vi "swerve_periodic.vi"(8 "Field Oriented?":bool, 9 "Rotate":dbl(slide) scale=-1.0..1.0, 10 "Forwards":dbl(slide) scale=-1.0..1.0, 11 "Strafe":dbl(slide) scale=-1.0..1.0) -> ()   [LabVIEW 2020]
uses:
  <vilib>/Rock Robotics/WPI/ThirdParty/Phoenix-LabVIEW/Motor Controller/Controls/CTRE_Phoenix_MotorControl_ControlMode.ctl
  swerve_globals.vi
  <vilib>/Rock Robotics/WPI/ThirdParty/Phoenix-LabVIEW/Motor Controller/Get/CTRE_Phoenix_MotorController_GetSelectedSensorData.vi
  TitanLib/Lib/TitanLib.lvlib
panel:
  in  "Set Constants":bool
  in  "Constants":T1
  out "Pose Estimation (in)":cluster{"Pose[0]":dbl, "Pose[1]":dbl}[](graph)
  in  "wheel offset (in)":dbl format="%_6g"
  in  "Reset Odometry?":bool
  in  "Drive Speed Multiplier":dbl=1.0
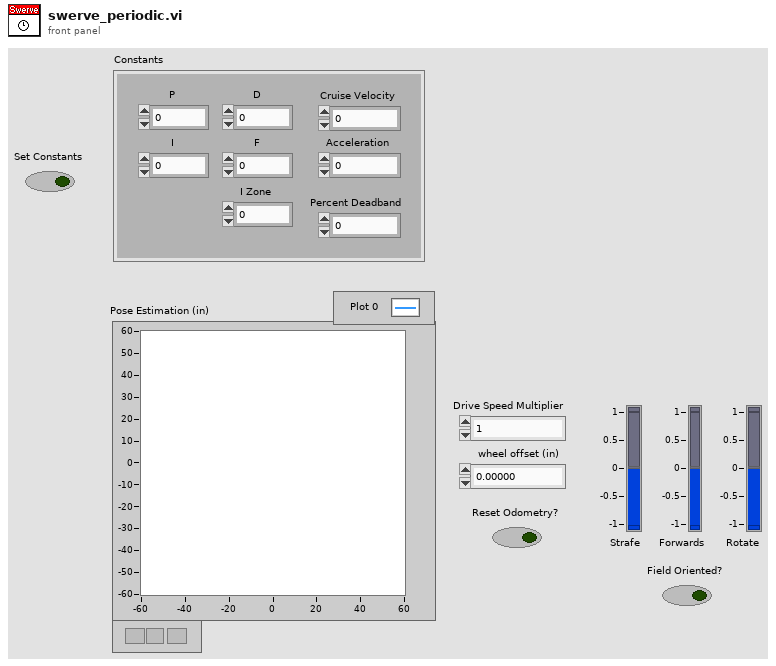
[diagram p1: front panel]
types:
  T1 = cluster{"P":dbl, "I":dbl, "D":dbl, "F":dbl, "I Zone":dbl, "Cruise Velocity":i32, "Acceleration":i32, "Percent Deadband":dbl}
  T2 = typedef "CTRE_Phoenix_MotorControl_ControlMode.ctl" = u16
  T3 = typedef "WPI_MotorControlDeviceRef.ctl" = cluster{"DeviceStatus":errorcluster, "Type":T4, "PWM":cluster{"PWM Channel":T5, "DeadBand":T6}, "CAN":cluster{"Device Number":u8, "SetOutput VI Ref":variant, "GetOutput VI Ref":variant, "Enable VI Ref":variant, "Disable VI Ref":variant, "Data":variant}, "Invert":bool, "DIO PWM":cluster{"PWM \"Enable\" Channel":T5, "DIOChannel":T7, "PWM Rate":dbl}}
  T4 = typedef "WPI_MotorControlType.ctl" = enum16{"PWM", "CAN", "DIO PWM"}
  T5 = typedef "FPGA_DIOPWMChannel.ctl" = enum8{"PWM 0", "PWM 1", "PWM 2", "PWM 3", "PWM 4", "PWM 5", "PWM 6", "PWM 7", "PWM 8", "PWM 9", "PWM MXP 0", "PWM MXP 1", "PWM MXP 2", "PWM MXP 3", "PWM MXP 4", "PWM MXP 5", "PWM MXP 6", "PWM MXP 7", "PWM MXP 8", "PWM MXP 9", "Invalid"}
  T6 = typedef "WPI_PWMDeadband.ctl" = cluster{"Name":string, "maxPositivePwm":i32, "minPositivePwm":i32, "centerPwm":i32, "maxNegativePwm":i32, "minNegativePwm":i32, "angularRange":u16}
  T7 = typedef "FPGA_DIOChannel.ctl" = enum8{"DIO 0", "DIO 1", "DIO 2", "DIO 3", "DIO 4", "DIO 5", "DIO 6", "DIO 7", "DIO 8", "DIO 9", "DIO MXP 0", "DIO MXP 1", "DIO MXP 2", "DIO MXP 3", "DIO MXP 4", "DIO MXP 5", "DIO MXP 6", "DIO MXP 7", "DIO MXP 8", "DIO MXP 9", "DIO MXP 10", "DIO MXP 11", "DIO MXP 12", "DIO MXP 13", "DIO MXP 14", "DIO MXP 15", "SPI Port CS1", "SPI Port CS2", "SPI Port CS3", "SPI Port MISO", "SPI Port MOSI", "Invalid"}
  T8 = typedef "NI_Matrix.lvlib/RealMatrix.ctl" = dbl[][]
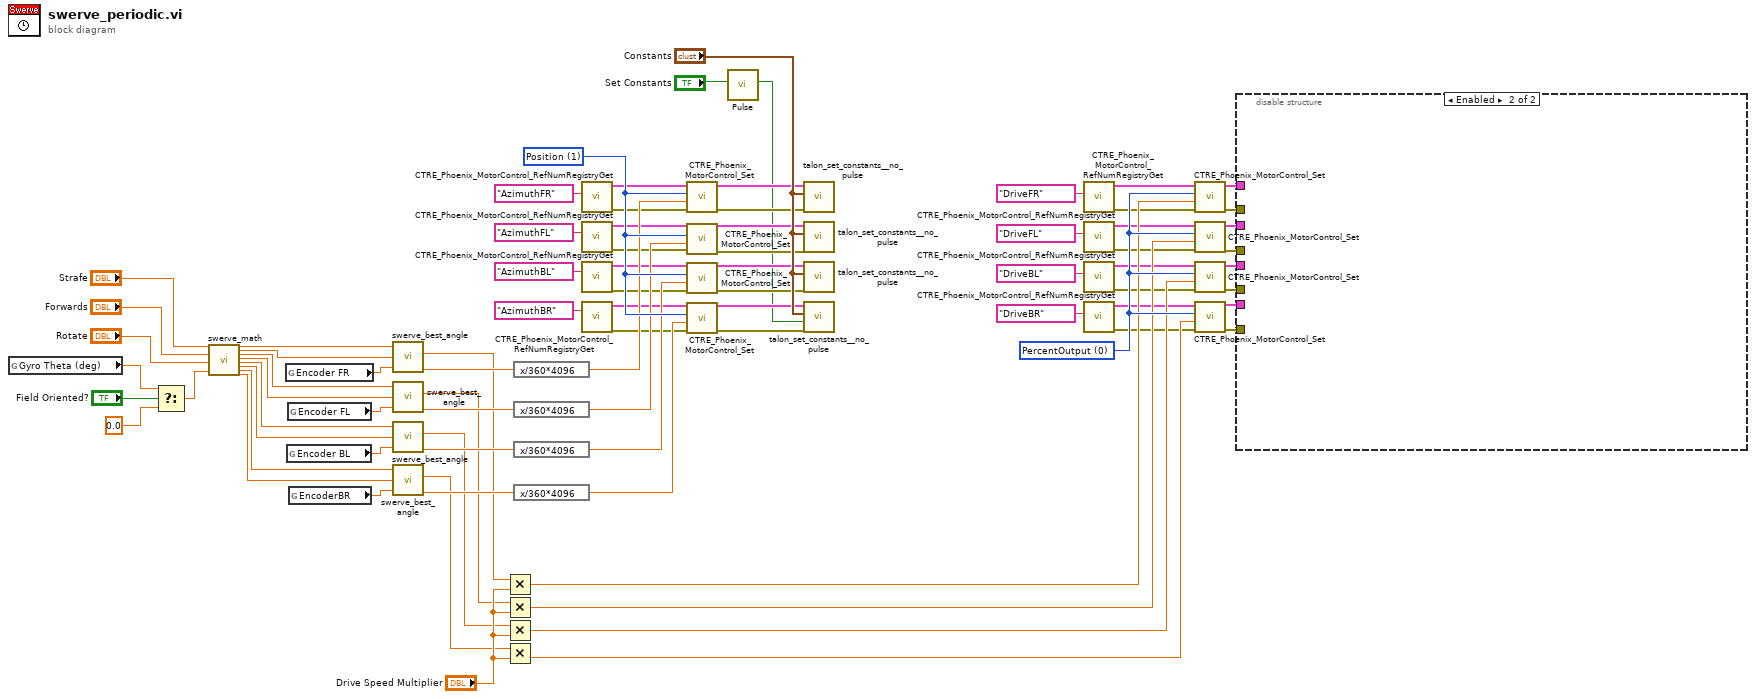
[diagram p0: block diagram]
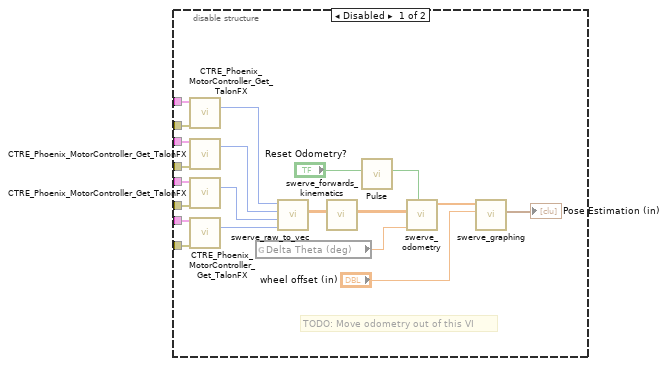
[diagram p2: hidden frame]
diagram:
  w67 = T2 0 items=["PercentOutput"=0, "Position"=1, "Velocity"=2, "Current"=3, "Follower"=5, "MotionProfile"=6, "MotionMagic"=7, "MotionProfileArc"=10, "Disabled"=15] ("Control Mode")
  w81 = T2 1 items=["PercentOutput"=0, "Position"=1, "Velocity"=2, "Current"=3, "Follower"=5, "MotionProfile"=6, "MotionMagic"=7, "MotionProfileArc"=10, "Disabled"=15] ("Control Mode")
  n1 = global read "swerve_globals.vi" "Gyro Theta (deg)"() -> (w18:dbl)
  n2 = Select(t=w18, s="Field Oriented?", f=0.0) -> (s? t:f=w16:dbl)
  n3 = call "swerve_math.vi"("Strafe"="Strafe", "Forwards"="Forwards", "Rotate"="Rotate", "Gyro"=w16) -> ("Drive FR"=w30:dbl, "Azimuth FR"=w25:dbl, "Drive FL"=w24:dbl, "Azimuth FL"=w23:dbl, "Drive BL"=w22:dbl, "Azimuth BL"=w21:dbl, "Drive BR"=w20:dbl, "Azimuth BR"=w19:dbl)  [unwired: 16 in]
  n4 = global read "swerve_globals.vi" "Encoder FR"() -> (w29:dbl)
  n5 = global read "swerve_globals.vi" "Encoder BL"() -> (w27:dbl)
  n6 = global read "swerve_globals.vi" "Encoder FL"() -> (w28:dbl)
  n7 = global read "swerve_globals.vi" "EncoderBR"() -> (w26:dbl)
  n8 = call "swerve_best_angle.vi"("Current Angle"=w29, "Target Angle"=w25, "Power In"=w30) -> ("Setpoint Angle"=w80:dbl, "Power Out"=w71:dbl)  [unwired: 4 in]
  n9 = call "swerve_best_angle.vi"("Current Angle"=w28, "Target Angle"=w23, "Power In"=w24) -> ("Setpoint Angle"=w79:dbl, "Power Out"=w70:dbl)  [unwired: 4 in]
  n10 = call "swerve_best_angle.vi"("Current Angle"=w27, "Target Angle"=w21, "Power In"=w22) -> ("Setpoint Angle"=w78:dbl, "Power Out"=w69:dbl)  [unwired: 4 in]
  n11 = call "swerve_best_angle.vi"("Current Angle"=w26, "Target Angle"=w19, "Power In"=w20) -> ("Setpoint Angle"=w77:dbl, "Power Out"=w68:dbl)  [unwired: 4 in]
  n12 = Multiply(x=w71, y="Drive Speed Multiplier") -> (x*y=w58:dbl)
  n13 = Multiply(x=w70, y="Drive Speed Multiplier") -> (x*y=w57:dbl)
  n14 = Multiply(x=w69, y="Drive Speed Multiplier") -> (x*y=w56:dbl)
  n15 = Multiply(x=w68, y="Drive Speed Multiplier") -> (x*y=w55:dbl)
  n16 = expression code="x/360*4096"(w80) -> (w76:dbl)
  n17 = expression code="x/360*4096"(w79) -> (w75:dbl)
  n18 = expression code="x/360*4096"(w78) -> (w74:dbl)
  n19 = expression code="x/360*4096"(w77) -> (w73:dbl)
  n20 = call <vilib>:"CTRE_Phoenix_MotorControl_RefNumRegistryGet.vi"("refnum name"="AzimuthFR") -> ("error out"=w49:errorcluster, "PhoenixMotorControlDevRef"=w50:T3)  [unwired: 9 in]
  n21 = call <vilib>:"CTRE_Phoenix_MotorControl_RefNumRegistryGet.vi"("refnum name"="AzimuthFL") -> ("error out"=w47:errorcluster, "PhoenixMotorControlDevRef"=w48:T3)  [unwired: 9 in]
  n22 = call <vilib>:"CTRE_Phoenix_MotorControl_RefNumRegistryGet.vi"("refnum name"="AzimuthBL") -> ("error out"=w45:errorcluster, "PhoenixMotorControlDevRef"=w46:T3)  [unwired: 9 in]
  n23 = call <vilib>:"CTRE_Phoenix_MotorControl_RefNumRegistryGet.vi"("refnum name"="AzimuthBR") -> ("error out"=w43:errorcluster, "PhoenixMotorControlDevRef"=w44:T3)  [unwired: 9 in]
  n24 = call <vilib>:"CTRE_Phoenix_MotorControl_Set.vi"("error in (no error)"=w49, "Output"=w76, "Control Mode"=w81, "PhoenixMotorControlDevRef"=w50) -> ("error out"=w9:errorcluster, "PhoenixMotorControlDevRef"=w10:T3)  [unwired: 6 in]
  n25 = call <vilib>:"CTRE_Phoenix_MotorControl_Set.vi"("error in (no error)"=w47, "Output"=w75, "Control Mode"=w81, "PhoenixMotorControlDevRef"=w48) -> ("error out"=w7:errorcluster, "PhoenixMotorControlDevRef"=w8:T3)  [unwired: 6 in]
  n26 = call <vilib>:"CTRE_Phoenix_MotorControl_Set.vi"("error in (no error)"=w45, "Output"=w74, "Control Mode"=w81, "PhoenixMotorControlDevRef"=w46) -> ("error out"=w5:errorcluster, "PhoenixMotorControlDevRef"=w6:T3)  [unwired: 6 in]
  n27 = call <vilib>:"CTRE_Phoenix_MotorControl_Set.vi"("error in (no error)"=w43, "Output"=w73, "Control Mode"=w81, "PhoenixMotorControlDevRef"=w44) -> ("error out"=w3:errorcluster, "PhoenixMotorControlDevRef"=w4:T3)  [unwired: 6 in]
  n28 = call "Pulse.vi"("Input"="Set Constants") -> ("Output"=w1:bool)  [unwired: 10 in]
  n29 = call "talon_set_constants__no_pulse.vi"("error in"=w9, "Constants"="Constants", "PhoenixMotorControlDevRef"=w10) -> ()  [unwired: 7 in, 2 out]
  n30 = call "talon_set_constants__no_pulse.vi"("error in"=w7, "Constants"="Constants", "PhoenixMotorControlDevRef"=w8) -> ()  [unwired: 7 in, 2 out]
  n31 = call "talon_set_constants__no_pulse.vi"("error in"=w5, "Constants"="Constants", "PhoenixMotorControlDevRef"=w6) -> ()  [unwired: 7 in, 2 out]
  n32 = call "talon_set_constants__no_pulse.vi"("error in"=w3, "Set Constants"=w1, "Constants"="Constants", "PhoenixMotorControlDevRef"=w4) -> ()  [unwired: 6 in, 2 out]
  n33 = call <vilib>:"CTRE_Phoenix_MotorControl_RefNumRegistryGet.vi"("refnum name"="DriveFR") -> ("error out"=w31:errorcluster, "PhoenixMotorControlDevRef"=w32:T3)  [unwired: 9 in]
  n34 = call <vilib>:"CTRE_Phoenix_MotorControl_RefNumRegistryGet.vi"("refnum name"="DriveFL") -> ("error out"=w33:errorcluster, "PhoenixMotorControlDevRef"=w34:T3)  [unwired: 9 in]
  n35 = call <vilib>:"CTRE_Phoenix_MotorControl_RefNumRegistryGet.vi"("refnum name"="DriveBL") -> ("error out"=w35:errorcluster, "PhoenixMotorControlDevRef"=w36:T3)  [unwired: 9 in]
  n36 = call <vilib>:"CTRE_Phoenix_MotorControl_RefNumRegistryGet.vi"("refnum name"="DriveBR") -> ("error out"=w37:errorcluster, "PhoenixMotorControlDevRef"=w38:T3)  [unwired: 9 in]
  n37 = call <vilib>:"CTRE_Phoenix_MotorControl_Set.vi"("error in (no error)"=w31, "Output"=w58, "Control Mode"=w67, "PhoenixMotorControlDevRef"=w32) -> ("error out"=w65:errorcluster, "PhoenixMotorControlDevRef"=w66:T3)  [unwired: 6 in]
  n38 = call <vilib>:"CTRE_Phoenix_MotorControl_Set.vi"("error in (no error)"=w33, "Output"=w57, "Control Mode"=w67, "PhoenixMotorControlDevRef"=w34) -> ("error out"=w63:errorcluster, "PhoenixMotorControlDevRef"=w64:T3)  [unwired: 6 in]
  n39 = call <vilib>:"CTRE_Phoenix_MotorControl_Set.vi"("error in (no error)"=w35, "Output"=w56, "Control Mode"=w67, "PhoenixMotorControlDevRef"=w36) -> ("error out"=w61:errorcluster, "PhoenixMotorControlDevRef"=w62:T3)  [unwired: 6 in]
  n40 = call <vilib>:"CTRE_Phoenix_MotorControl_Set.vi"("error in (no error)"=w37, "Output"=w55, "Control Mode"=w67, "PhoenixMotorControlDevRef"=w38) -> ("error out"=w59:errorcluster, "PhoenixMotorControlDevRef"=w60:T3)  [unwired: 6 in]
  n41 = disable-structure shown="Enabled" {
    disable-tunnel: w66 -> [w101 _]
    disable-tunnel: w65 -> [w100 _]
    disable-tunnel: w64 -> [w99 _]
    disable-tunnel: w63 -> [w98 _]
    disable-tunnel: w62 -> [w97 _]
    disable-tunnel: w61 -> [w96 _]
    disable-tunnel: w60 -> [w95 _]
    disable-tunnel: w59 -> [w94 _]
    frame Disabled {
      # "TODO: Move odometry out of this VI"
      n42 = call-poly <vilib>:"CTRE_Phoenix_MotorController_Get_TalonFX.vi"("PhoenixMotorControlDevRef"=w101, "error in"=w100) -> ("Position (Raw Sensor Units)"=w92:i32)  [unwired: 10 in, 3 out]
      n43 = call-poly <vilib>:"CTRE_Phoenix_MotorController_Get_TalonFX.vi"("PhoenixMotorControlDevRef"=w99, "error in"=w98) -> ("Position (Raw Sensor Units)"=w91:i32)  [unwired: 10 in, 3 out]
      n44 = call-poly <vilib>:"CTRE_Phoenix_MotorController_Get_TalonFX.vi"("PhoenixMotorControlDevRef"=w97, "error in"=w96) -> ("Position (Raw Sensor Units)"=w90:i32)  [unwired: 10 in, 3 out]
      n45 = call-poly <vilib>:"CTRE_Phoenix_MotorController_Get_TalonFX.vi"("PhoenixMotorControlDevRef"=w95, "error in"=w94) -> ("Position (Raw Sensor Units)"=w85:i32)  [unwired: 10 in, 3 out]
      n46 = global read "swerve_globals.vi" "Delta Theta (deg)"() -> (w86:dbl)
      n47 = call "swerve_raw_to_vec.vi"("Raw Position BR"=w85, "Raw Position BL"=w90, "Raw Position FL"=w91, "Raw Position FR"=w92) -> ("Output Vector"=w84:T8)  [unwired: 7 in]
      n48 = call "swerve_forwards_kinematics.vi"("Input Vector"=w84) -> ("Output Vector"=w89:T8)  [unwired: 10 in]
      n49 = call "Pulse.vi"("Input"="Reset Odometry?") -> ("Output"=w82:bool)  [unwired: 10 in]
      n50 = call "swerve_odometry.vi"("Reset?"=w82, "Delta Theta (deg)"=w86, "input vector"=w89) -> ("Pose"=w88:dbl[])  [unwired: 8 in]
      n51 = call "swerve_graphing.vi"("wheel offset"="wheel offset (in)", "Pose"=w88) -> ("Output"=→"Pose Estimation (in)":cluster{"x out":dbl, "y out":dbl}[])  [unwired: 9 in]
    }
    frame Enabled {
    }
  }
